vi "startIVAndWait.vi"(8 "error in (no error)":errorcluster, 11 "Instrument.Lockin in":refnum<class "Instrument.Lockin.lvclass">) -> (0 "error out":errorcluster, 2 "AI Waveform":waveform(dbl)[](array[waveform]), 3 "Instrument.Lockin out":refnum<class "Instrument.Lockin.lvclass">)   [LabVIEW 2019, in "Instrument.Lockin.lvclass"]
uses:
  Instrument.Lockin.lvclass
panel:
  in  "stop":bool
  out "timer (s)":dbl=1.2239999771118164
  # "This VI triggers the lockin and waits until the acquisition is complete"
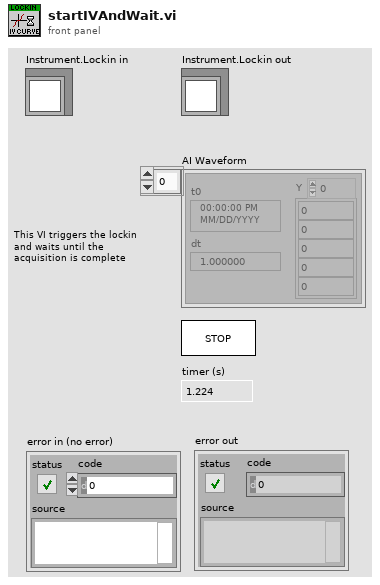
[diagram p1: front panel]
types:
  T1 = typedef "Lockin.DAQ.lvclass/AO-cluster.ctl" = T2[]
  T2 = typedef "Instrument.Lockin.UI.lvclass/AO Channel--Cluster.ctl" = cluster{"Enable?":bool, "Channel":i32, "Amplitude":dbl, "Offset":dbl, "Frequency":dbl, "Phase":dbl, "Function":T3, "Sweeping?":bool}
  T3 = typedef "Lockin.DAQ.lvclass/Function-enum.ctl" = enum16{"Sine", "Triangle", "Square"}
  T4 = typedef "Lockin.DAQ.lvclass/State-enum.ctl" = enum16{"idle", "created", "started", "stopped", "sweeping"}
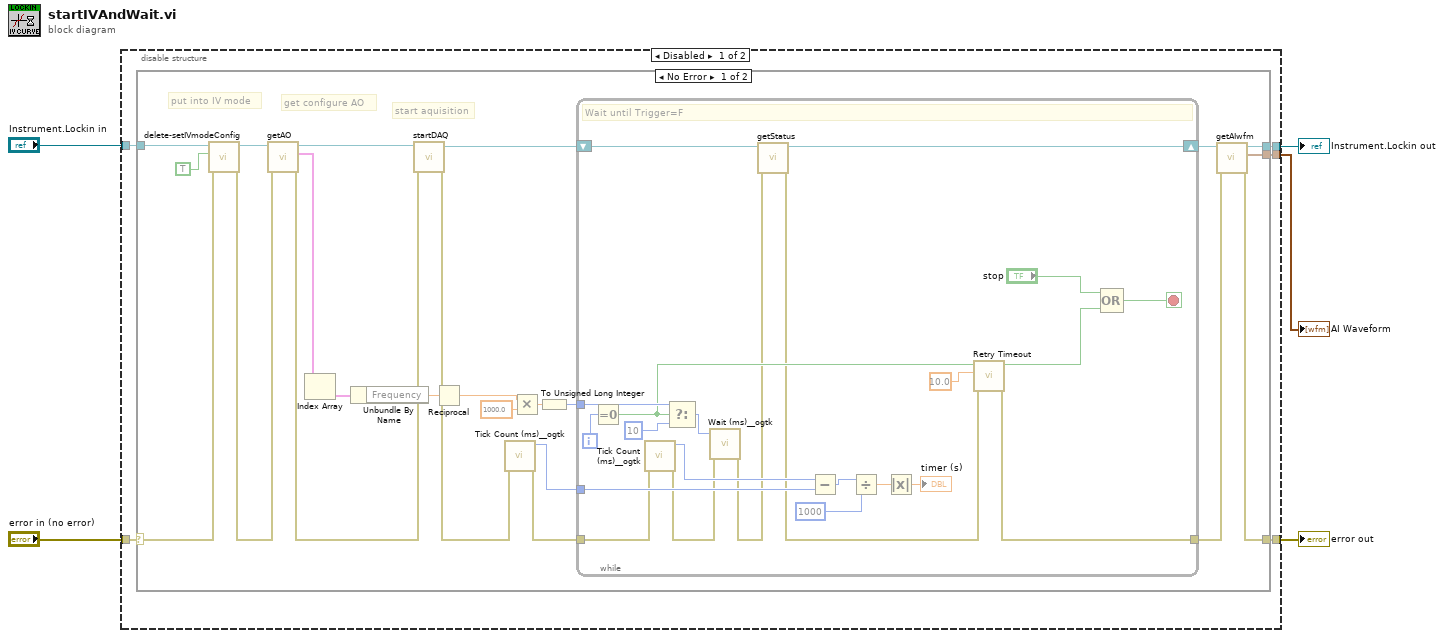
[diagram p0: block diagram]
diagram:
  n1 = disable-structure shown="Disabled" {
    disable-tunnel: [w10 _] -> w5
    disable-tunnel: [w9 _] -> w4
    disable-tunnel: "Instrument.Lockin in" -> [w8 _]
    disable-tunnel: [w7 _] -> w2
    disable-tunnel: "error in (no error)" -> [w6 _]
    frame Disabled {
      n2 = case shown="No Error" w6 {
        selector: w6 -> [w17 w59]
        tunnel: [w14 w59] -> w10
        tunnel: [w28 _] -> w9
        tunnel: w8 -> [w18 w58]
        tunnel: [w19 w58] -> w7
        frame No Error {
          # "start aquisition"
          # "get configure AO"
          # "put into IV mode"
          n3 = call "delete-setIVmodeConfig.vi"("error in (no error)"=w17, "IV mode"=TRUE, "Instrument.Lockin in"=w18) -> ("error out"=w24:errorcluster, "Instrument.Lockin out"=w23:refnum<class "Instrument.Lockin.lvclass">)  [unwired: 7 in]
          n4 = call "getAO.vi"("error in (no error)"=w24, "Instrument.Lockin in"=w23) -> ("error out"=w22:errorcluster, "AOconfig"=w13:T1, "Instrument.Lockin out"=w21:refnum<class "Instrument.Lockin.lvclass">)  [unwired: 7 in]
          n5 = Index Array(array=w13) -> (element=w12:T2)  [unwired: 1 in]
          n6 = Unbundle By Name(w12) -> ("Frequency"=w11:dbl)
          n7 = call "startDAQ.vi"("error in (no error)"=w22, "Instrument.Lockin in"=w21) -> ("error out"=w20:errorcluster, "Instrument.Lockin out"=w26:refnum<class "Instrument.Lockin.lvclass">)  [unwired: 8 in]
          n8 = Reciprocal(x=w11) -> (1/x=w30:dbl)
          n9 = call <userlib>:"Tick Count (ms)__ogtk.vi"("error in (no error)"=w20) -> ("error out"=w16:errorcluster, "millisecond timer value"=w33:u32)  [unwired: 9 in]
          n10 = Multiply(x=w30, y=1000.0) -> (x*y=w31:dbl)
          n11 = To Unsigned Long Integer(number=w31) -> (unsigned 32bit integer=w29:u32)
          n12 = while {
            tunnel: w33 -> [w55]
            tunnel: w29 -> [w50]
            tunnel: w16 -> [w41]
            tunnel: [w40] -> w15
            shift-right: [w48] -> w27
            shift-left: w26 -> [w47]
            i -> [w52]
            stop <- w54 stop-if-true
            # "Wait until Trigger=F"
            n13 = Equal To 0?(x=w52) -> (x = 0?=w43:bool)
            n14 = call <userlib>:"Tick Count (ms)__ogtk.vi"("error in (no error)"=w41) -> ("error out"=w53:errorcluster, "millisecond timer value"=w56:u32)  [unwired: 9 in]
            n15 = Select(t=w50, s=w43, f=u32 10) -> (s? t:f=w51:u32)
            n16 = call <userlib>:"Wait (ms)__ogtk.vi"("error in (no error)"=w53, "milliseconds to wait"=w51) -> ("error out"=w38:errorcluster)  [unwired: 8 in, 1 out]
            n17 = call "getStatus.vi"("error in (no error)"=w38, "Instrument.Lockin"=w47) -> ("error out"=w39:errorcluster, "Status"=w49:T4, "Instrument.Lockin"=w48:refnum<class "Instrument.Lockin.lvclass">)  [unwired: 7 in]
            n18 = Subtract(x=w56, y=w55) -> (x-y=w44:u32)
            n19 = Divide(x=w44, y=u32 1000 ("x")) -> (x/y=w46:dbl)
            n20 = Absolute Value(x=w46) -> (abs(x)=→"timer (s)":dbl)
            n21 = call "Retry Timeout.vi"("error in (no error)"=w39, "time (s) [10 s]"=10.0, "reset"=w43) -> ("error out"=w40:errorcluster, "Timeout?"=w35:bool)  [unwired: 7 in]
            n22 = Compound Arithmetic op=OR("stop", w35) -> (w54:bool, w37:bool)
          }
          n23 = call "getAIwfm.vi"("error in (no error)"=w15, "Instrument.Lockin in"=w27) -> ("error out"=w14:errorcluster, "AI Waveform"=w28:waveform(dbl)[], "Instrument.Lockin out"=w19:refnum<class "Instrument.Lockin.lvclass">)  [unwired: 7 in]
        }
        frame Error {
        }
      }
    }
    frame Enabled {
    }
  }
  "error out" <- w5
  "AI Waveform" <- w4
  "Instrument.Lockin out" <- w2
